vi "New SenseHat.vi"(8 "error in (no error)":errorcluster, 11 "LINX Resource":T1) -> (0 "error out":errorcluster, 3 "SenseHat out":refnum<class "SenseHat.lvclass">)   [LabVIEW 2020, in "RPI.SenseHat.lvlib" / "SenseHat.lvclass"]
uses:
  SenseHat.lvclass
  <vilib>/MakerHub/LINX/Private/Type Defs/LINX Ref.ctl
  <vilib>/MakerHub/LINX/Private/Type Defs/Platform.ctl
  <vilib>/MakerHub/LINX/Private/Type Defs/Interface.ctl
  <vilib>/MakerHub/LINX/Private/Device/Type Defs/LINX Device Config.ctl
  <vilib>/MakerHub/LINX/Private/Device/Type Defs/TCP Config.ctl
  <vilib>/MakerHub/LINX/Private/Device/Type Defs/Channels.ctl
  SenseHat.lvclass/SenseHat.ctl
  RPI/Classes/mainI2CDevice/mainI2CDevice.lvclass
  <vilib>/MakerHub/LINX/LMH-LINX.lvlib
  <vilib>/MakerHub/LINX/Private/Device/Device.lvlib
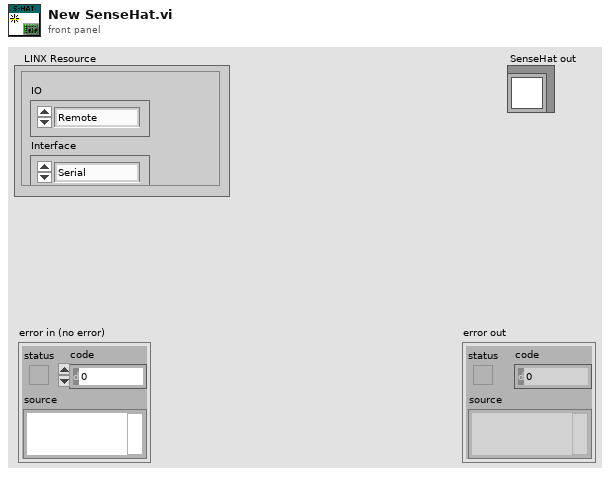
[diagram p1: front panel]
types:
  T1 = typedef "LMH-LINX.lvlib/LINX Ref.ctl" = cluster{"IO":T2, "Interface":T3, "LINX Device Config":T4}
  T2 = typedef "LMH-LINX.lvlib/Platform.ctl" = enum16{"Remote", "Local"}
  T3 = typedef "LMH-LINX.lvlib/Interface.ctl" = enum16{"Serial", "TCP"}
  T4 = typedef "LMH-LINX.lvlib/Device.lvlib/LINX Device Config.ctl" = cluster{"Interface":T3, "COM Port":refnum<visa-resource-name>, "TCP Configuration":T5, "Device Family":u8, "Device ID":u8, "Device Name":string, "TCP Ref":refnum<k5>, "Channels":T6}
  T5 = typedef "LMH-LINX.lvlib/Device.lvlib/TCP Config.ctl" = cluster{"IP Address":string, "Port":u16}
  T6 = typedef "LMH-LINX.lvlib/Channels.ctl" = cluster{"DI":u8[], "DO":u8[], "AI":u8[], "AO":u8[], "PWM":u8[], "QE":u8[], "UART":u8[], "I2C 2":u8[], "SPI":u8[], "CAN":u8[], "Servo":u8[], "AI Ref (V)":dbl, "AI Resolution (Bits)":u8, "AO Ref (V)":dbl, "AO Resolution (Bits)":u8}
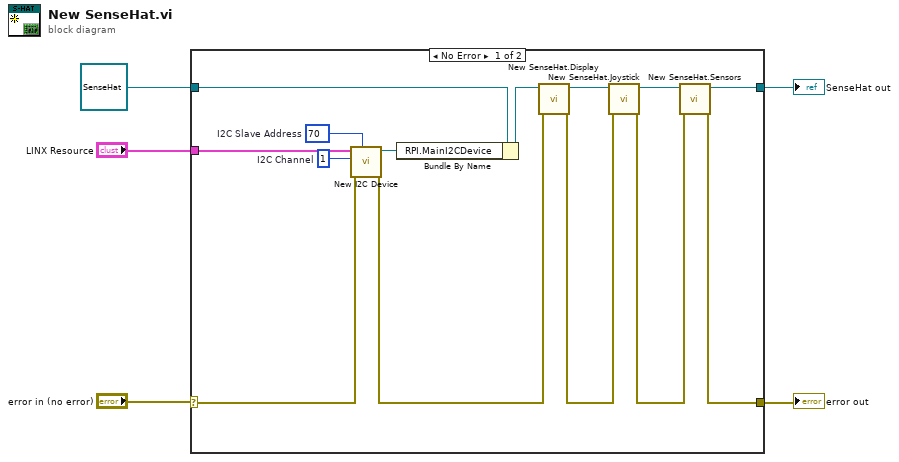
[diagram p0: block diagram]
diagram:
  n1 = case shown="No Error" "error in (no error)" {
    selector: "error in (no error)" -> [w15 w20]
    tunnel: refnum<class "SenseHat.lvclass"> refnum ("SenseHat in") -> [w19 w21]
    tunnel: [w8 w21] -> w4
    tunnel: [w6 w20] -> w2
    tunnel: "LINX Resource" -> [w18 _]
    frame No Error {
      w16 = u8 1  # I2C Channel
      w17 = u8 70  # I2C Slave Address
      n2 = call "New I2C Device.vi"("I2C Slave Address"=w17, "error in (no error)"=w15, "I2C Channel"=w16, "object in"=w18) -> ("error out"=w12:errorcluster, "mainI2CDevice out"=w14:refnum<class "mainI2CDevice.lvclass">)  [unwired: 6 in]
      n3 = Bundle By Name(cluster=w19, "RPI.MainI2CDevice"=w14) -> (w13:refnum<class "SenseHat.lvclass">)
      n4 = call "New SenseHat.Display.vi"("error in (no error)"=w12, "SenseHat in"=w13) -> ("error out"=w10:errorcluster, "SenseHat out"=w11:refnum<class "SenseHat.lvclass">)  [unwired: 8 in]
      n5 = call "New SenseHat.Joystick.vi"("error in (no error)"=w10, "SenseHat in"=w11) -> ("error out"=w7:errorcluster, "SenseHat out"=w9:refnum<class "SenseHat.lvclass">)  [unwired: 8 in]
      n6 = call "New SenseHat.Sensors.vi"("error in (no error)"=w7, "SenseHat in"=w9) -> ("error out"=w6:errorcluster, "SenseHat out"=w8:refnum<class "SenseHat.lvclass">)  [unwired: 8 in]
    }
    frame Error {
    }
  }
  "SenseHat out" <- w4
  "error out" <- w2
